vi "PNAclose.vi"(1 "Error In (no error)":errorcluster, 2 "VISA session":refnum<visa-resource-name>) -> (0 "Error Out":errorcluster)   [LabVIEW 2017]
uses:
  <instrlib>/Agilent PNA Series/Agilent PNA Series.lvlib
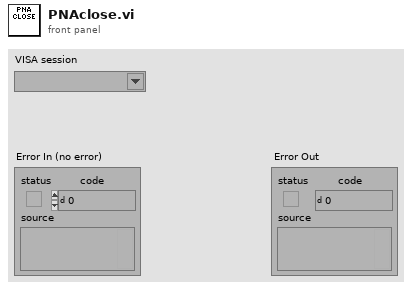
[diagram p1: front panel]
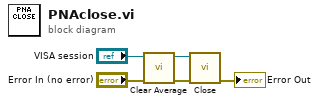
[diagram p0: block diagram]
diagram:
  n1 = call <instrlib>:"Clear Average.vi"("Error In (no error)"="Error In (no error)", "VISA Resource Name"="VISA session") -> ("Error Out"=w4:errorcluster, "VISA Resource Name Out"=w5:refnum<visa-resource-name>)  [unwired: 8 in]
  n2 = call <instrlib>:"Close.vi"("Error In (no error)"=w4, "VISA Resource Name"=w5) -> ("Error Out"=→"Error Out":errorcluster)  [unwired: 9 in]
